vi "Zero.vi"() -> ()   [LabVIEW 2013]
panel:
  in  "Zero":dbl
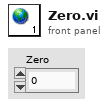
[diagram p1: front panel]
diagram:
